vi "ErrorLog_BuildFilePaths.vi"(8 "error in (no error)":errorcluster, 11 "reference in":refnum<class "ErrorLog.lvclass">) -> (0 "error out":errorcluster, 3 "reference out":refnum<class "ErrorLog.lvclass">)   [LabVIEW 2017, in "ErrorLog.lvclass"]
uses:
  ErrorLog.lvclass
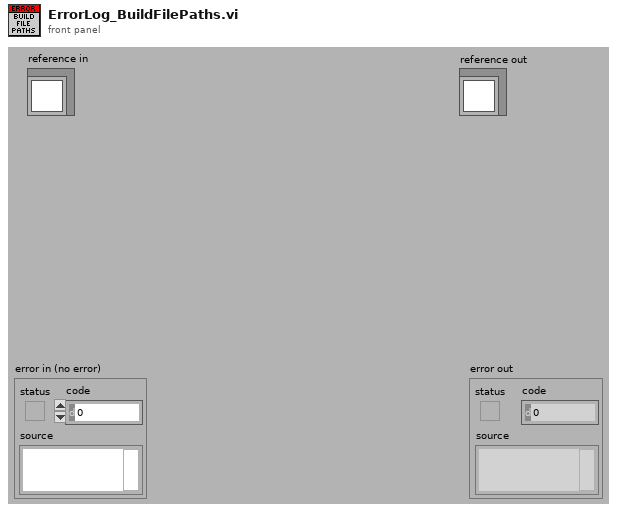
[diagram p1: front panel]
types:
  T1 = typedef "ErrorLog.lvclass/ObjectAttributes.ctl" = cluster{"ErrorFile":path, "Supress Consecutive Duplicates":bool, "Errors":string, "Quit":bool, "Errors since last call":string, "Last Recorded Error":string, "ErrorPath":path, "PossiblePaths":path[], "BaseFileName":string, "Max Log Files":i32, "ErrorFile Index":i32, "Max File Size":i64}
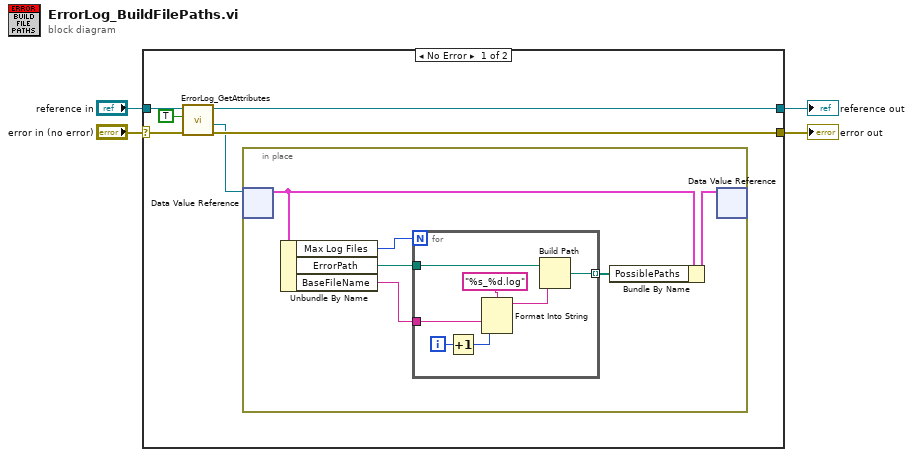
[diagram p0: block diagram]
diagram:
  n1 = case shown="No Error" "error in (no error)" {
    selector: "error in (no error)" -> [w10 w25]
    tunnel: [w9 w25] -> w3
    tunnel: [w7 w24] -> w1
    tunnel: "reference in" -> [w8 w24]
    frame No Error {
      n2 = call "ErrorLog_GetAttributes.vi"("error in (no error)"=w10, "OnlyGetDvrReference(False)"=TRUE, "reference in"=w8) -> ("error out"=w9:errorcluster, "DataRef"=w5:refnum<data-value>, "reference out"=w7:refnum<class "ErrorLog.lvclass">)  [unwired: 5 in, 1 out]
      n3 = in-place {
        n4 = in-place-dvr #1(w5) -> (w14:T1)  [unwired: 1 out]
        n5 = Unbundle By Name(w14) -> ("Max Log Files"=w11:i32, "ErrorPath"=w15:path, "BaseFileName"=w16:string)
        n6 = for {
          N: w11 -> [_]
          tunnel: w15 -> [w23]
          tunnel: w16 -> [w22]
          tunnel: [w17] -> w13 mode=indexing
          i -> [w21]
          n7 = Increment(x=w21) -> (x+1=w20:i32)
          n8 = Format Into String(format string="%s_%d.log" ("name or relative path"), w22, w20) -> (resulting string=w19:string)  [unwired: 2 in, 1 out]
          n9 = Build Path(base path=w23, name or relative path=w19) -> (appended path=w17:path)
        }
        n10 = Bundle By Name(cluster=w14, "PossiblePaths"=w13) -> (w12:T1)
        n11 = in-place-dvr #1(w12) -> ()  [unwired: 2 out]
      }
    }
    frame Error {
    }
  }
  "error out" <- w3
  "reference out" <- w1
